vi "Is status ongoing - string.vi"(1 "Monkey Status":string) -> (0 "Monkey Running?":bool)   [LabVIEW 2020]
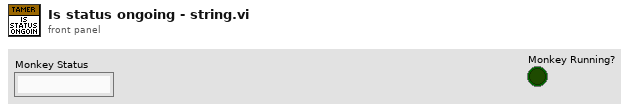
[diagram p1: front panel]
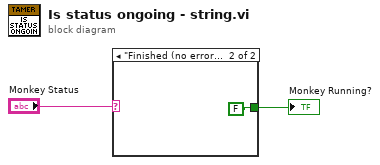
[diagram p0: block diagram]
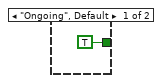
[diagram p2: hidden frame]
diagram:
  n1 = case shown="\"Finished (no errors)\", \"Finished (with errors)\", \"Stopped\"" "Monkey Status" {
    tunnel: [TRUE FALSE] -> w1
    frame "Ongoing", Default {
    }
    frame "Finished (no errors)", "Finished (with errors)", "Stopped" {
    }
  }
  "Monkey Running?" <- w1
